vi "Read Config.vi"() -> (0 "error out":errorcluster)   [LabVIEW 2020]
panel:
  in  "Names":string[](array[string])=["PRODUCT_ID", "HARDWARE_VERSION", "FIRMWARE_VERSION", "BOOTLOADER_VERSION", "WIFI_VERSION", "SERIAL_NUMBER", "POWER_ETHERNET_DEFAULT", "POWER_WIFI_DEFAULT", "POWER_AIN_DEFAULT", "POWER_LED_DEFAULT"]
  out "Error String":string
  out "ConnectionType Out":i32
  out "DeviceType Out":i32
  in  "Identifier":string="LJM_idANY"
  in  "ConnectionType":string="LJM_ctANY"
  in  "DeviceType":string="LJM_dtANY"
  out "Values":dbl[](array[numeric]) format="%.4f"
  out "ErrorAddress":i32
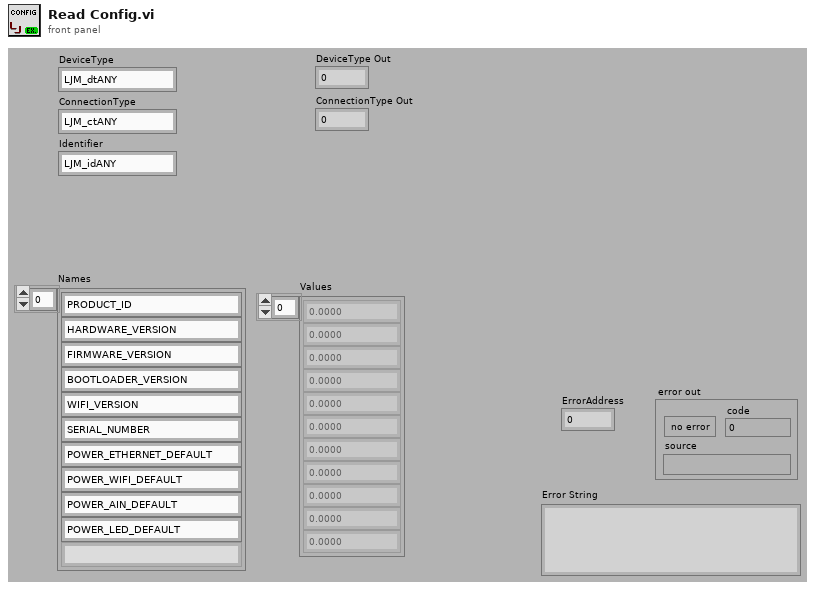
[diagram p1: front panel]
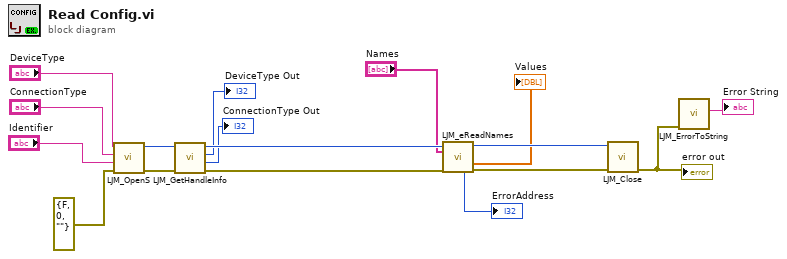
[diagram p0: block diagram]
diagram:
  n1 = call "LJM_OpenS.vi"("error in"=errorcluster {"status"=FALSE, "code"=0, "source"=""} ("error in (no error)"), "Identifier"="Identifier", "ConnectionType"="ConnectionType", "DeviceType"="DeviceType") -> ("error out"=w15:errorcluster, "Handle"=w13:i32)  [unwired: 6 in]
  n2 = call "LJM_GetHandleInfo.vi"("error in"=w15, "Handle In"=w13) -> ("error out"=w14:errorcluster, "ConnectionType"=→"ConnectionType Out":i32, "DeviceType"=→"DeviceType Out":i32, "Handle Out"=w12:i32)  [unwired: 2 in, 4 out]
  n3 = call "LJM_eReadNames.vi"("Handle In"=w12, "aNames"="Names", "error in"=w14) -> ("Handle Out"=w11:i32, "aValuesOut"=→"Values":dbl[], "ErrorAddress"=→"ErrorAddress":i32, "error out"=w16:errorcluster)  [unwired: 9 in]
  n4 = call "LJM_Close.vi"("error in"=w16, "Handle"=w11) -> ("error out"=w5:errorcluster)  [unwired: 9 in]
  "error out" <- w5
  n5 = call "LJM_ErrorToString.vi"("error in"=w5) -> ("String"=→"Error String":string)  [unwired: 10 in]
